vi "Keep Angle.vi"(8 "Angle":dbl, 9 "Right Speed":dbl, 10 "Left Speed":dbl, 11 "Keep Angle":bool) -> (1 "Right":dbl, 2 "Left":dbl)   [LabVIEW 2016]
uses:
  <vilib>/addons/control/pid/pid.llb/PID (DBL).vi
  <vilib>/addons/control/pid/NI_PID_pid.lvlib
panel:
  in  "PID gains":T1={"proportional gain (Kc)"=0.05, "integral time (Ti, min)"=0.0, "derivative time (Td, min)"=0.0}
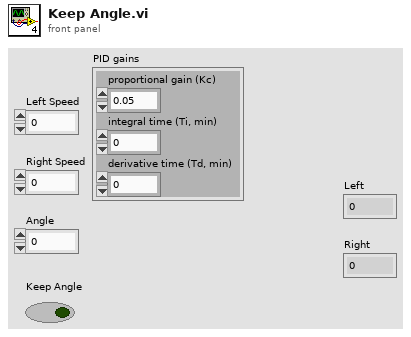
[diagram p1: front panel]
types:
  T1 = cluster{"proportional gain (Kc)":dbl, "integral time (Ti, min)":dbl, "derivative time (Td, min)":dbl}
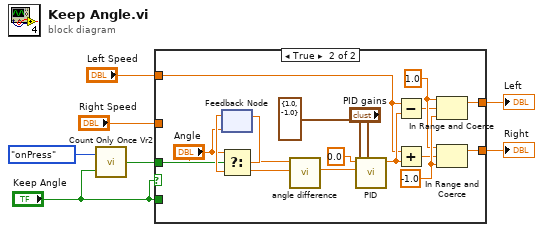
[diagram p0: block diagram]
diagram:
  n1 = call "Count Only Once Vr2.vi"("InValue"="Keep Angle", "Action"=enum16{"onPress", "onRelease", "Both"}."onPress") -> ("Result"=w1:bool)
  n2 = case shown="True" "Keep Angle" {
    tunnel: [w9 w17] -> w7
    tunnel: [w8 w16] -> w6
    tunnel: "Keep Angle" -> [_ _]
    tunnel: "Left Speed" -> [w9 w15]
    tunnel: "Right Speed" -> [w8 _]
    tunnel: w1 -> [_ w14]
    frame False {
    }
    frame True {
      w22 = -1.0 ("lower limit")
      w21 = 1.0 ("upper limit")
      n3 = feedback #1("Angle") -> (w25:dbl)
      n4 = Select(t="Angle", s=w14, f=w25) -> (s? t:f=w13:dbl)
      n5 = feedback-in #1(w13) -> ()
      n6 = call "angle difference.vi"("angle2"=w13, "angle1"="Angle") -> ("angle diff"=w23:dbl)  [unwired: 9 in]
      n7 = call-poly <vilib>:"PID.vi"("output range"=cluster{"output high":dbl, "output low":dbl} {"output high"=1.0, "output low"=-1.0}, "PID gains"="PID gains", "process variable"=w23, "setpoint"=0.0) -> ("output"=w19:dbl)  [unwired: 6 in, 1 out]
      n8 = Subtract(x=w15, y=w19) -> (x-y=w20:dbl)
      n9 = Add(x=w15, y=w19) -> (x+y=w18:dbl)
      n10 = In Range and Coerce(upper limit=w21, x=w20, lower limit=w22) -> (coerced(x)=w17:dbl)  [unwired: 1 out]
      n11 = In Range and Coerce(upper limit=w21, x=w18, lower limit=w22) -> (coerced(x)=w16:dbl)  [unwired: 1 out]
    }
  }
  "Left" <- w7
  "Right" <- w6
